vi "log analysis_gps.vi"() -> ()   [LabVIEW 2018] (continued)
\n\t\n15:48:12.2\tlog_raw\tgps_raw\t\tsystem status\tnormal 2 27.700000 0 0\trobot status\t93.017900\t121.985005\t8.053800\t-0.255095\t0.011947\t-127.616619\t0.344000\t0.011000\n\t\n15:48:12.7\tlog_raw\tgps_raw\t\tsystem status\tnormal 2 27.700000 0 0\trobot status\t92.936548\t121.892392\t8.053400\t-0.560051\t-0.370997\t-128.619129\t0.179000\t-0.036000\n\t\n15:48:13.2\tlog_raw\tgps_raw\t\tsystem status\tnormal 2 27.600000 0 0\trobot status\t92.838145\t121.787255\t8.053000\t-0.462743\t-0.497171\t-129.892844\t0.237000\t-0.153000\n\t\n15:48:13.7\tlog_raw\tgps_raw\t#INSPVAXA,USB3,0,46.5,FINESTEERING,2107,283711.750,02000000,471d,15824;INS_ALIGNMENT_COMPLETE,INS_RTKFIXED,37.37122661325,126.72188206330,8.0523,22.3000,-0.1946,-0.1990,0.0081,-0.343732019,-0.465256456,221.217414786,0.4342,0.3030,0.5793,0.1138,0.0937,0.0785,0.0954,0.0993,5.0883,0f000001,0*d2ab07a9\n\tsystem status\tnormal 2 27.600000 0 0\trobot status\t92.737843\t121.684862\t8.052300\t-0.343732\t-0.465256\t-131.217415\t0.296000\t-0.048000\n\t\n15:48:14.2\tlog_raw\tgps_raw\t#INSPVAXA,USB3,0,44.5,FINESTEERING,2107,283712.250,02000000,471d,15824;INS_ALIGNMENT_COMPLETE,INS_RTKFIXED,37.37122571809,126.72188087797,8.0513,22.3000,-0.1877,-0.2276,0.0316,0.179753839,-0.491470448,222.605830014,0.4342,0.3024,0.5794,0.1134,0.0940,0.0785,0.0954,0.0992,5.0887,0f000001,0*82158439\n\tsystem status\tnormal 2 27.500000 0 0\trobot status\t92.632849\t121.585514\t8.051300\t0.179754\t-0.491470\t-132.605830\t0.302000\t-0.060000\n\t\n15:48:14.7\tlog_raw\tgps_raw\t\tsystem status\tnormal 2 27.500000 0 0\trobot status\t92.530950\t121.487165\t8.046000\t-0.221044\t-0.411824\t-134.007632\t0.276000\t-0.043000\n\t\n15:48:15.2\tlog_raw\tgps_raw\t\tsystem status\tnormal 2 27.600000 0 0\trobot status\t92.422232\t121.387491\t8.042500\t-0.513663\t-0.512668\t-135.162406\t0.345000\t0.039000\n\t\n15:48:15.7\tlog_raw\tgps_raw\t\tsystem status\tnormal 2 27.600000 0 0\trobot status\t92.311835\t121.294033\t8.039900\t-0.332842\t-0.481399\t-136.078923\t0.343000\t0.036000\n\t\n15:48:16.2\tlog_raw\tgps_raw\t\tsystem status\tnormal 2 27.700000 0 0\trobot status\t92.199321\t121.200404\t8.038800\t-0.246424\t-0.569738\t-136.851756\t0.285000\t-0.056000\n\t\n15:48:16.7\tlog_raw\tgps_raw\t\tsystem status\tnormal 2 27.700000 0 0\trobot status\t92.091706\t121.109962\t8.035500\t-0.515195\t-0.354482\t-137.596544\t0.302000\t0.015000\n\t\n15:48:17.2\tlog_raw\tgps_raw\t\tsystem status\tnormal 2 27.800000 0 0\trobot status\t91.984102\t121.023401\t8.032900\t-0.648117\t-0.096859\t-138.155271\t0.305000\t0.062000\n\t\n15:48:17.7\tlog_raw\tgps_raw\t#INSPVAXA,USB3,0,49.5,FINESTEERING,2107,283715.750,02000000,471d,15824;INS_ALIGNMENT_COMPLETE,INS_RTKFIXED,37.37122004093,126.72187255202,8.0310,22.3000,-0.2525,-0.3284,0.0150,-0.722312377,-0.111566034,228.459144624,0.4339,0.3022,0.5793,0.1124,0.0928,0.0785,0.0954,0.0992,5.0842,0f000001,0*1d534d62\n\tsystem status\tnormal 2 27.700000 0 0\trobot status\t91.895350\t120.955445\t8.031000\t-0.722312\t-0.111566\t-138.459145\t0.356000\t0.005000\n\t\n15:48:18.2\tlog_raw\tgps_raw\t\tsystem status\tnormal 2 27.800000 0 0\trobot status\t91.784347\t120.867609\t8.027400\t-0.870891\t-0.276065\t-138.775579\t0.323000\t0.011000\n\t\n15:48:18.7\tlog_raw\tgps_raw\t\tsystem status\tnormal 2 27.800000 0 0\trobot status\t91.667786\t120.777478\t8.023500\t-0.860571\t-0.105772\t-139.137030\t0.415000\t0.024000\n\t\n15:48:19.2\tlog_raw\tgps_raw\t\tsystem status\tnormal 2 27.800000 0 0\trobot status\t91.467289\t120.615612\t8.019000\t-1.126128\t-0.570366\t-139.574346\t0.506000\t0.026000\n\t\n15:48:19.7\tlog_raw\tgps_raw\t\tsystem status\tnormal 2 27.900000 0 0\trobot status\t91.290630\t120.476156\t8.013000\t-1.186175\t-0.952521\t-139.872615\t0.485000\t0.025000\n\t\n15:48:20.2\tlog_raw\tgps_raw\t\tsystem status\tnormal 2 27.800000 0 0\trobot status\t91.107922\t120.338579\t8.010700\t-0.902776\t-1.033275\t-140.087143\t0.506000\t0.009000\n\t\n15:48:20.7\tlog_raw\tgps_raw\t\tsystem status\tnormal 2 27.800000 0 0\trobot status\t90.917995\t120.193959\t8.006900\t-1.049748\t-0.623872\t-140.229198\t0.504000\t0.022000\n\t\n15:48:21.2\tlog_raw\tgps_raw\t\tsystem status\tnormal 2 27.800000 0 0\trobot status\t90.727645\t120.053075\t8.003300\t-1.012052\t-0.230090\t-140.363200\t0.489000\t0.034000\n\t\n15:48:21.7\tlog_raw\tgps_raw\t\tsystem status\tnormal 2 27.800000 0 0\trobot status\t90.535348\t119.912993\t8.001800\t-0.988290\t-0.249157\t-140.250323\t0.490000\t0.034000\n\t\n15:48:22.2\tlog_raw\tgps_raw\t\tsystem status\tnormal 2 27.800000 0 0\trobot status\t90.365162\t119.792234\t7.999800\t-0.881256\t-0.195383\t-140.162244\t0.439000\t-0.029000\n\t\n15:48:22.7\tlog_raw\tgps_raw\t\tsystem status\tnormal 2 27.700000 0 0\trobot status\t90.166459\t119.645467\t7.997200\t-0.990730\t-0.386708\t-139.693095\t0.448000\t0.064000\n\t\n15:48:23.2\tlog_raw\tgps_raw\t\tsystem status\tnormal 2 27.600000 0 0\trobot status\t89.980110\t119.505285\t7.995900\t-0.920399\t-0.411056\t-138.884517\t0.331000\t0.293000\n\t\n15:48:23.7\tlog_raw\tgps_raw\t\tsystem status\tnormal 2 27.500000 0 0\trobot status\t89.798925\t119.364391\t7.991900\t-0.934473\t-0.125823\t-137.685217\t0.780000\t-0.350000\n\t\n15:48:24.3\tlog_raw\tgps_raw\t\tsystem status\tnormal 2 27.500000 0 0\trobot status\t89.618396\t119.217719\t7.990900\t-0.955434\t-0.178314\t-136.420655\t0.729000\t-0.315000\n\t\n15:48:24.8\tlog_raw\tgps_raw\t\tsystem status\tnormal 2 27.500000 0 0\trobot status\t89.438061\t119.065932\t7.990300\t-0.897105\t-0.363562\t-134.936703\t0.627000\t-0.123000\n\t\n15:48:25.3\tlog_raw\tgps_raw\t\tsystem status\tnormal 2 27.500000 0 0\trobot status\t89.259742\t118.908481\t7.988300\t-0.702072\t-0.768658\t-133.619038\t0.555000\t-0.042000\n\t\n15:48:25.8\tlog_raw\tgps_raw\t\tsystem status\tnormal 2 27.500000 0 0\trobot status\t89.085735\t118.748193\t7.985800\t-0.541349\t-0.915935\t-132.332460\t0.561000\t-0.086000\n\t\n15:48:26.3\tlog_raw\tgps_raw\t\tsystem status\tnormal 2 27.500000 0 0\trobot status\t88.921991\t118.588618\t7.982500\t-0.622601\t-0.502395\t-131.080219\t0.355000\t0.255000\n\t\n15:48:26.8\tlog_raw\tgps_raw\t\tsystem status\tnormal 2 27.500000 0 0\trobot status\t88.757318\t118.422538\t7.979600\t-0.531381\t-0.385527\t-129.950730\t0.648000\t-0.197000\n\t\n15:48:27.3\tlog_raw\tgps_raw\t\tsystem status\tnormal 2 27.500000 0 0\trobot status\t88.594631\t118.254427\t7.977200\t-0.446190\t-0.411819\t-128.968277\t0.666000\t-0.210000\n\t\n15:48:27.8\tlog_raw\tgps_raw\t\tsystem status\tnormal 2 27.600000 0 0\trobot status\t88.436524\t118.081442\t7.976100\t-0.854908\t-0.480169\t-128.206928\t0.457000\t0.071000\n\t\n15:48:28.3\tlog_raw\tgps_raw\t\tsystem status\tnormal 2 27.600000 0 0\trobot status\t88.280978\t117.911050\t7.973300\t-0.840223\t-0.485683\t-127.350658\t0.578000\t-0.111000\n\t\n15:48:28.8\tlog_raw\tgps_raw\t\tsystem status\tnormal 2 27.600000 0 0\trobot status\t88.125157\t117.734701\t7.973300\t-0.975629\t-0.460087\t-126.734726\t0.581000\t-0.092000\n\t\n15:48:29.3\tlog_raw\tgps_raw\t\tsystem status\tnormal 2 27.700000 0 0\trobot status\t87.972781\t117.556566\t7.972400\t-1.249899\t-0.684709\t-126.312420\t0.395000\t0.153000\n\t\n15:48:29.8\tlog_raw\tgps_raw\t\tsystem status\tnormal 2 27.700000 0 0\trobot status\t87.818562\t117.377164\t7.971600\t-1.130025\t-0.574230\t-125.881307\t0.422000\t0.152000\n\t\n15:48:30.3\tlog_raw\tgps_raw\t\tsystem status\tnormal 2 27.700000 0 0\trobot status\t87.670351\t117.200299\t7.971700\t-1.245931\t-0.391971\t-125.531082\t0.668000\t-0.259000\n\t\n15:48:30.8\tlog_raw\tgps_raw\t\tsystem status\tnormal 2 27.700000 0 0\trobot status\t87.521983\t117.020319\t7.971300\t-1.373248\t0.023524\t-125.204569\t0.362000\t0.195000\n\t\n15:48:31.3\tlog_raw\tgps_raw\t\tsystem status\tnormal 2 27.700000 0 0\trobot status\t87.374479\t116.840408\t7.972200\t-1.262386\t0.158447\t-124.787590\t0.497000\t0.002000\n\t\n15:48:31.8\tlog_raw\tgps_raw\t\tsystem status\tnormal 2 27.700000 0 0\trobot status\t87.236829\t116.671092\t7.974200\t-1.228214\t0.108580\t-124.545435\t0.542000\t0.007000\n\t\n15:48:32.3\tlog_raw\tgps_raw\t\tsystem status\tnormal 2 27.700000 0 0\trobot status\t87.089765\t116.488767\t7.975900\t-1.256331\t-0.129864\t-124.336401\t0.483000\t0.032000\n\t\n15:48:32.8\tlog_raw\tgps_raw\t\tsystem status\tnormal 2 27.700000 0 0\trobot status\t86.942897\t116.305166\t7.980600\t-1.436628\t0.013062\t-124.042497\t0.592000\t-0.138000\n\t\n15:48:33.3\tlog_raw\tgps_raw\t\tsystem status\tnormal 2 27.700000 0 0\trobot status\t86.791583\t116.117809\t7.982400\t-1.131604\t-0.146521\t-123.890554\t0.459000\t0.013000\n\t\n15:48:33.8\tlog_raw\tgps_raw\t#INSPVAXA,USB3,0,50.0,FINESTEERING,2107,283731.800,02000000,471d,15824;INS_ALIGNMENT_COMPLETE,INS_RTKFIXED,37.37117458679,126.72181307353,7.9818,22.3000,-0.3273,-0.2857,0.0109,-1.190065034,-0.069687290,213.721334289,0.4352,0.3028,0.5840,0.1128,0.0931,0.0809,0.0959,0.1000,5.0570,0f000001,0*9dfc8b18\n\tsystem status\tnormal 2 27.700000 0 0\trobot status\t86.626842\t115.910791\t7.981800\t-1.190065\t-0.069687\t-123.721334\t0.413000\t0.130000\n\t\n15:48:34.3\tlog_raw\tgps_raw\t\tsystem status\tnormal 2 27.800000 0 0\trobot status\t86.494276\t115.741589\t7.984700\t-1.380691\t-0.163770\t-123.599724\t0.490000\t0.027000\n\t\n15:48:34.8\tlog_raw\tgps_raw\t#INSPVAXA,USB3,0,51.0,FINESTEERING,2107,283732.800,02000000,471d,15824;INS_ALIGNMENT_COMPLETE,INS_RTKFIXED,37.37117121797,126.72180974634,7.9878,22.3000,-0.3313,-0.2857,0.0219,-1.270635454,-0.215524516,213.339771314,0.4352,0.3028,0.5846,0.1129,0.0933,0.0811,0.0960,0.1001,5.0551,0f000001,0*0aee9a35\n\tsystem status\tnormal 2 27.700000 0 0\trobot status\t86.332125\t115.536907\t7.987800\t-1.270635\t-0.215525\t-123.339771\t0.555000\t-0.092000\n\t\n15:48:35.3\tlog_raw\tgps_raw\t#INSPVAXA,USB3,0,51.5,FINESTEERING,2107,283733.300,02000000,471d,15824;INS_ALIGNMENT_COMPLETE,INS_RTKFIXED,37.37116954427,126.72180813326,7.9908,22.3000,-0.3552,-0.2859,0.0156,-1.448481440,-0.233169639,213.103409582,0.4350,0.3026,0.5849,0.1127,0.0932,0.0807,0.0961,0.1001,5.0540,0f000001,0*6eded770\n\tsystem status\tnormal 2 27.700000 0 0\trobot status\t86.189241\t115.351153\t7.990800\t-1.448481\t-0.233170\t-123.103410\t0.418000\t0.134000\n\t\n15:48:35.8\tlog_raw\tgps_raw\t\tsystem status\tnormal 2 27.700000 0 0\trobot status\t86.059476\t115.180486\t7.992600\t-1.482871\t-0.440891\t-122.862305\t0.381000\t0.175000\n\t\n15:48:36.3\tlog_raw\tgps_raw\t#INSPVAXA,USB3,0,50.5,FINESTEERING,2107,283734.300,02000000,471d,15824;INS_ALIGNMENT_COMPLETE,INS_RTKFIXED,37.37116643278,126.72180513242,7.9941,22.3000,-0.3478,-0.2920,-0.0081,-1.453049667,-0.445591431,212.491210472,0.4347,0.3023,0.5850,0.1126,0.0932,0.0804,0.0961,0.1001,5.0539,0f000001,0*79c2ad3a\n\tsystem status\tnormal 2 27.700000 0 0\trobot status\t85.923432\t115.005828\t7.994100\t-1.453050\t-0.445591\t-122.491210\t0.407000\t0.062000\n\t\n15:48:36.8\tlog_raw\tgps_raw\t\tsystem status\tnormal 2 27.700000 0 0\trobot status\t85.785092\t114.822258\t7.996500\t-1.200019\t-0.747046\t-122.371203\t0.383000\t0.098000\n\t\n15:48:37.3\tlog_raw\tgps_raw\t\tsystem status\tnormal 2 27.800000 0 0\trobot status\t85.644286\t114.630005\t7.999900\t-1.162405\t-0.500187\t-122.112655\t0.546000\t-0.078000\n\t\n15:48:37.8\tlog_raw\tgps_raw\t#INSPVAXA,USB3,0,50.0,FINESTEERING,2107,283735.800,02000000,471d,15824;INS_ALIGNMENT_COMPLETE,INS_RTKFIXED,37.37116119506,126.72180032977,8.0024,22.3000,-0.3542,-0.2959,0.0116,-1.070253035,-0.077101790,211.926024212,0.4346,0.3023,0.5850,0.1127,0.0933,0.0801,0.0962,0.1001,5.0543,0f000001,0*c680b455\n\tsystem status\tnormal 2 27.700000 0 0\trobot status\t85.498021\t114.424526\t8.002400\t-1.070253\t-0.077102\t-121.926024\t0.603000\t-0.154000\n\t\n15:48:38.3\tlog_raw\tgps_raw\t#INSPVAXA,USB3,0,52.5,FINESTEERING,2107,283736.300,02000000,471d,15824;INS_ALIGNMENT_COMPLETE,INS_RTKFIXED,37.37115947932,126.72179880714,8.0040,22.3000,-0.3644,-0.2930,0.0272,-1.158322238,-0.026079764,211.769815237,0.4340,0.3014,0.5849,0.1129,0.0936,0.0802,0.0962,0.1001,5.0557,0f000001,0*91878766\n\tsystem status\tnormal 2 27.700000 0 0\trobot status\t85.363149\t114.234107\t8.004000\t-1.158322\t-0.026080\t-121.769815\t0.444000\t0.091000\n\t\n15:48:38.8\tlog_raw\tgps_raw\t\tsystem status\tnormal 2 27.700000 0 0\trobot status\t85.241349\t114.062655\t8.007800\t-1.147952\t0.031214\t-121.613966\t0.431000\t0.095000\n\t\n15:48:39.3\tlog_raw\tgps_raw\t#INSPVAXA,USB3,0,49.5,FINESTEERING,2107,283737.300,02000000,471d,15824;INS_ALIGNMENT_COMPLETE,INS_RTKFIXED,37.37115601705,126.72179575213,8.0111,22.3000,-0.3535,-0.2715,0.0236,-1.072991275,-0.157444358,211.337264747,0.4338,0.3020,0.5848,0.1128,0.0935,0.0799,0.0962,0.1000,5.0571,0f000001,0*fcfec35c\n\tsystem status\tnormal 2 27.700000 0 0\trobot status\t85.092541\t113.849851\t8.011100\t-1.072991\t-0.157444\t-121.337265\t0.639000\t-0.209000\n\t\n15:48:39.8\tlog_raw\tgps_raw\t#INSPVAXA,USB3,0,49.5,FINESTEERING,2107,283737.800,02000000,471d,15824;INS_ALIGNMENT_COMPLETE,INS_RTKFIXED,37.37115424403,126.72179422575,8.0146,22.3000,-0.3686,-0.2725,0.0313,-1.104138059,-0.177331016,211.359293731,0.4338,0.3020,0.5848,0.1128,0.0935,0.0799,0.0962,0.1000,5.0571,0f000001,0*ab5647ea\n\tsystem status\tnormal 2 27.800000 0 0\trobot status\t84.957337\t113.653075\t8.014600\t-1.104138\t-0.177331\t-121.359294\t0.430000\t0.099000\n\t\n15:48:40.3\tlog_raw\tgps_raw\t\tsystem status\tnormal 2 27.700000 0 0\trobot status\t84.838628\t113.477755\t8.016900\t-1.353747\t-0.132621\t-121.323522\t0.573000\t-0.118000\n\t\n15:48:40.8\tlog_raw\tgps_raw\t\tsystem status\tnormal 2 27.800000 0 0\trobot status\t84.707094\t113.291580\t8.018800\t-1.250301\t-0.380341\t-121.163525\t0.339000\t-0.018000\n\t\n15:48:41.3\tlog_raw\tgps_raw\t#INSPVAXA,USB3,0,49.5,FINESTEERING,2107,283739.300,02000000,471d,15824;INS_ALIGNMENT_COMPLETE,INS_RTKFIXED,37.37114934907,126.72178999234,8.0211,22.3000,-0.4739,-0.3464,0.0176,-1.136581936,-0.167253224,210.967892029,0.4333,0.3019,0.5842,0.1128,0.0941,0.0795,0.0961,0.1000,5.0600,0f000001,0*70943433\n\tsystem status\tnormal 2 27.700000 0 0\trobot status\t84.582348\t113.109813\t8.021100\t-1.136582\t-0.167253\t-120.967892\t0.521000\t0.039000\n\t\n15:48:41.8\tlog_raw\tgps_raw\t\tsystem status\tnormal 2 27.800000 0 0\trobot status\t84.470112\t112.943563\t8.022300\t-1.050765\t-0.308716\t-120.878935\t0.430000\t0.006000\n\t\n15:48:42.3\tlog_raw\tgps_raw\t\tsystem status\tnormal 2 27.800000 0 0\trobot status\t84.332743\t112.735829\t8.022200\t-1.089765\t-0.132879\t-120.991930\t0.485000\t0.008000\n\t\n15:48:42.8\tlog_raw\tgps_raw\t#INSPVAXA,USB3,0,50.0,FINESTEERING,2107,283740.800,02000000,471d,15824;INS_ALIGNMENT_COMPLETE,INS_RTKFIXED,37.37114414583,126.72178561946,8.0225,22.3000,-0.3822,-0.2779,0.0042,-1.093019003,-0.010151528,210.947598498,0.4332,0.3033,0.5839,0.1127,0.0932,0.0793,0.0961,0.0999,5.0603,0f000001,0*1136f991\n\tsystem status\tnormal 2 27.700000 0 0\trobot status\t84.195006\t112.532337\t8.022500\t-1.093019\t-0.010152\t-120.947598\t0.504000\t0.001000\n\t\n15:48:43.3\tlog_raw\tgps_raw\t\tsystem status\tnormal 2 27.800000 0 0\trobot status\t84.075902\t112.352166\t8.023600\t-1.338722\t-0.304524\t-121.104447\t0.480000\t-0.009000\n\t\n15:48:43.8\tlog_raw\tgps_raw\t#INSPVAXA,USB3,0,48.5,FINESTEERING,2107,283741.800,02000000,471d,15824;INS_ALIGNMENT_COMPLETE,INS_RTKFIXED,37.37114058594,126.72178265531,8.0253,22.3000,-0.3567,-0.2593,0.0215,-1.513936100,-0.057286463,211.372668569,0.4332,0.3024,0.5836,0.1132,0.0938,0.0801,0.0960,0.0999,5.0615,0f000001,0*2f761fac\n\tsystem status\tnormal 2 27.800000 0 0\trobot status\t83.932446\t112.137247\t8.025300\t-1.513936\t-0.057286\t-121.372669\t0.502000\t-0.009000\n\t\n15:48:44.3\tlog_raw\tgps_raw\t#INSPVAXA,USB3,0,48.5,FINESTEERING,2107,283742.300,02000000,471d,15824;INS_ALIGNMENT_COMPLETE,INS_RTKFIXED,37.37113883610,126.72178116483,8.0251,22.3000,-0.3566,-0.2646,-0.0002,-1.629553261,-0.371874785,211.544863069,0.4334,0.3022,0.5834,0.1130,0.0935,0.0799,0.0960,0.0999,5.0629,0f000001,0*db798f34\n\tsystem status\tnormal 2 27.800000 0 0\trobot status\t83.800422\t111.943043\t8.025100\t-1.629553\t-0.371875\t-121.544863\t0.489000\t-0.014000\n\t\n15:48:44.8\tlog_raw\tgps_raw\t#INSPVAXA,USB3,0,48.5,FINESTEERING,2107,283742.800,02000000,471d,15824;INS_ALIGNMENT_COMPLETE,INS_RTKFIXED,37.37113713184,126.72177968059,8.0243,22.3000,-0.3489,-0.2579,0.0216,-1.473854332,-0.365287327,211.722184950,0.4334,0.3022,0.5834,0.1130,0.0935,0.0799,0.0960,0.0999,5.0629,0f000001,0*7daa81b7\n\tsystem status\tnormal 2 27.800000 0 0\trobot status\t83.668950\t111.753898\t8.024300\t-1.473854\t-0.365287\t-121.722185\t0.486000\t-0.016000\n\t\n15:48:45.3\tlog_raw\tgps_raw\t#INSPVAXA,USB3,0,46.0,FINESTEERING,2107,283743.300,02000000,471d,15824;INS_ALIGNMENT_COMPLETE,INS_RTKFIXED,37.37113541318,126.72177817924,8.0241,22.3000,-0.3602,-0.2594,0.0280,-1.547897785,-0.197369444,211.857866163,0.4337,0.3019,0.5833,0.1132,0.0937,0.0803,0.0960,0.0999,5.0644,0f000001,0*9acc447f\n\tsystem status\tnormal 2 27.800000 0 0\trobot status\t83.535963\t111.563154\t8.024100\t-1.547898\t-0.197369\t-121.857866\t0.490000\t-0.018000\n\t\n15:48:45.8\tlog_raw\tgps_raw\t#INSPVAXA,USB3,0,46.0,FINESTEERING,2107,283743.800,02000000,471d,15824;INS_ALIGNMENT_COMPLETE,INS_RTKFIXED,37.37113371860,126.72177667415,8.0236,22.3000,-0.3426,-0.2605,-0.0024,-1.484785571,-0.050192547,211.992358658,0.4337,0.3019,0.5833,0.1132,0.0937,0.0803,0.0960,0.0999,5.0644,0f000001,0*53a396a3\n\tsystem status\tnormal 2 27.800000 0 0\trobot status\t83.402645\t111.375083\t8.023600\t-1.484786\t-0.050193\t-121.992359\t0.494000\t-0.016000\n\t\n15:48:46.3\tlog_raw\tgps_raw\t#INSPVAXA,USB3,0,49.5,FINESTEERING,2107,283744.300,02000000,471d,15824;INS_ALIGNMENT_COMPLETE,INS_RTKFIXED,37.37113201879,126.72177513465,8.0232,22.3000,-0.3446,-0.2615,0.0259,-1.383371091,0.074969047,212.298273108,0.4337,0.3020,0.5833,0.1129,0.0934,0.0801,0.0960,0.0999,5.0660,0f000001,0*aa113718\n\tsystem status\tnormal 2 27.800000 0 0\trobot status\t83.266279\t111.186432\t8.023200\t-1.383371\t0.074969\t-122.298273\t0.499000\t-0.007000\n\t\n15:48:46.8\tlog_raw\tgps_raw\t#INSPVAXA,USB3,0,49.5,FINESTEERING,2107,283744.800,02000000,471d,15824;INS_ALIGNMENT_COMPLETE,INS_RTKFIXED,37.37113032635,126.72177358354,8.0234,22.3000,-0.3375,-0.2772,0.0273,-1.329281946,0.043160679,212.609113265,0.4337,0.3020,0.5833,0.1129,0.0934,0.0801,0.0960,0.0999,5.0660,0f000001,0*0ee78c5b\n\tsystem status\tnormal 2 27.800000 0 0\trobot status\t83.128884\t110.998599\t8.023400\t-1.329282\t0.043161\t-122.609113\t0.489000\t-0.016000\n\t\n15:48:47.3\tlog_raw\tgps_raw\t#INSPVAXA,USB3,0,52.0,FINESTEERING,2107,283745.300,02000000,471d,15824;INS_ALIGNMENT_COMPLETE,INS_RTKFIXED,37.37112862779,126.72177199929,8.0231,22.3000,-0.3459,-0.2782,0.0216,-1.184506207,0.212511857,212.764446314,0.4334,0.3022,0.5833,0.1126,0.0933,0.0799,0.0960,0.0999,5.0673,0f000001,0*6b47a2c0\n\tsystem status\tnormal 2 27.800000 0 0\trobot status\t82.988553\t110.810086\t8.023100\t-1.184506\t0.212512\t-122.764446\t0.506000\t-0.008000\n\t\n15:48:47.8\tlog_raw\tgps_raw\t\tsystem status\tnormal 2 27.800000 0 0\trobot status\t82.860769\t110.640040\t8.024500\t-1.218748\t0.257104\t-123.000230\t0.493000\t-0.007000\n\t\n15:48:48.3\tlog_raw\tgps_raw\t#INSPVAXA,USB3,0,50.5,FINESTEERING,2107,283746.300,02000000,471d,15824;INS_ALIGNMENT_COMPLETE,INS_RTKFIXED,37.37112521282,126.72176875566,8.0246,22.3000,-0.3436,-0.2866,0.0107,-1.152398634,0.173487967,213.302028541,0.4332,0.3024,0.5833,0.1125,0.0932,0.0797,0.0960,0.0999,5.0684,0f000001,0*49aabec8\n\tsystem status\tnormal 2 27.800000 0 0\trobot status\t82.701238\t110.431080\t8.024600\t-1.152399\t0.173488\t-123.302029\t0.485000\t-0.005000\n\t\n15:48:48.8\tlog_raw\tgps_raw\t#INSPVAXA,USB3,0,50.5,FINESTEERING,2107,283746.800,02000000,471d,15824;INS_ALIGNMENT_COMPLETE,INS_RTKFIXED,37.37112349330,126.72176709470,8.0242,22.3000,-0.3497,-0.2797,0.0191,-1.314916766,0.110853537,213.600359109,0.4332,0.3024,0.5833,0.1125,0.0932,0.0797,0.0960,0.0999,5.0684,0f000001,0*7436a872\n\tsystem status\tnormal 2 27.800000 0 0\trobot status\t82.554113\t110.240241\t8.024200\t-1.314917\t0.110854\t-123.600359\t0.500000\t-0.013000\n\t\n15:48:49.3\tlog_raw\tgps_raw\t#INSPVAXA,USB3,0,49.0,FINESTEERING,2107,283747.300,02000000,471d,15824;INS_ALIGNMENT_COMPLETE,INS_RTKFIXED,37.37112180863,126.72176542630,8.0244,22.3000,-0.3486,-0.2973,0.0020,-1.259459400,-0.205839817,213.873121305,0.4330,0.3028,0.5834,0.1123,0.0929,0.0795,0.0961,0.0999,5.0687,0f000001,0*73ffb7ee\n\tsystem status\tnormal 2 27.800000 0 0\trobot status\t82.406329\t110.053270\t8.024400\t-1.259459\t-0.205840\t-123.873121\t0.501000\t-0.018000\n\t\n15:48:49.8\tlog_raw\tgps_raw\t#INSPVAXA,USB3,0,49.0,FINESTEERING,2107,283747.800,02000000,471d,15824;INS_ALIGNMENT_COMPLETE,INS_RTKFIXED,37.37112013539,126.72176372884,8.0242,22.3000,-0.3447,-0.2936,0.0201,-1.219688710,-0.227511135,214.058949387,0.4330,0.3028,0.5834,0.1123,0.0929,0.0795,0.0961,0.0999,5.0687,0f000001,0*4b57b427\n\tsystem status\tnormal 2 27.800000 0 0\trobot status\t82.255971\t109.867567\t8.024200\t-1.219689\t-0.227511\t-124.058949\t0.493000\t-0.003000\n\t\n15:48:50.3\tlog_raw\tgps_raw\t\tsystem status\tnormal 2 27.800000 0 0\trobot status\t82.125100\t109.705360\t8.022900\t-1.272959\t-0.391336\t-124.294640\t0.474000\t0.015000\n\t\n15:48:50.8\tlog_raw\tgps_raw\t#INSPVAXA,USB3,0,51.0,FINESTEERING,2107,283748.800,02000000,471d,15824;INS_ALIGNMENT_COMPLETE,INS_RTKFIXED,37.37111693523,126.72176047327,8.0217,22.3000,-0.3794,-0.3424,0.0221,-1.127145988,-0.211560747,214.369143208,0.4328,0.3022,0.5832,0.1125,0.0931,0.0797,0.0961,0.0999,5.0695,0f000001,0*f768fbb4\n\tsystem status\tnormal 2 27.800000 0 0\trobot status\t81.967598\t109.512402\t8.021700\t-1.127146\t-0.211561\t-124.369143\t0.521000\t0.000000\n\t\n15:48:51.3\tlog_raw\tgps_raw\t#INSPVAXA,USB3,0,48.0,FINESTEERING,2107,283749.300,02000000,471d,15824;INS_ALIGNMENT_COMPLETE,INS_RTKFIXED,37.37111528295,126.72175880850,8.0228,22.3000,-0.3091,-0.2843,0.0017,-1.226699576,0.077786636,214.515601245,0.4326,0.3019,0.5831,0.1128,0.0935,0.0801,0.0961,0.1000,5.0707,0f000001,0*33e38593\n\tsystem status\tnormal 2 27.800000 0 0\trobot status\t81.820135\t109.329026\t8.022800\t-1.226700\t0.077787\t-124.515601\t0.481000\t-0.012000\n\t\n15:48:51.8\tlog_raw\tgps_raw\t#INSPVAXA,USB3,0,48.0,FINESTEERING,2107,283749.800,02000000,471d,15824;INS_ALIGNMENT_COMPLETE,INS_RTKFIXED,37.37111354772,126.72175702907,8.0230,22.3000,-0.3442,-0.3142,0.0177,-1.011041502,-0.010822308,214.650851385,0.4326,0.3019,0.5831,0.1128,0.0935,0.0801,0.0961,0.1000,5.0707,0f000001,0*157ce5bb\n\tsystem status\tnormal 2 27.800000 0 0\trobot status\t81.662516\t109.136443\t8.023000\t-1.011042\t-0.010822\t-124.650851\t0.501000\t0.006000\n\t\n15:48:52.3\tlog_raw\tgps_raw\t\tsystem status\tnormal 2 27.800000 0 0\trobot status\t81.529444\t108.971054\t8.023600\t-1.134131\t-0.000127\t-124.709887\t0.497000\t0.000000\n\t\n15:48:52.8\tlog_raw\tgps_raw\t\tsystem status\tnormal 2 27.800000 0 0\trobot status\t81.377778\t108.780675\t8.026800\t-1.391204\t-0.015262\t-124.810162\t0.496000\t0.005000\n\t\n15:48:53.3\tlog_raw\tgps_raw\t#INSPVAXA,USB3,0,50.0,FINESTEERING,2107,283751.300,02000000,471d,15824;INS_ALIGNMENT_COMPLETE,INS_RTKFIXED,37.37110849817,126.72175192105,8.0275,22.3000,-0.3358,-0.3126,0.0172,-1.035437411,0.273015584,214.819783864,0.4328,0.3018,0.5834,0.1129,0.0936,0.0806,0.0961,0.1000,5.0732,0f000001,0*f034d66d\n\tsystem status\tnormal 2 27.800000 0 0\trobot status\t81.210056\t108.576025\t8.027500\t-1.035437\t0.273016\t-124.819784\t0.503000\t-0.001000\n\t\n15:48:53.8\tlog_raw\tgps_raw\t#INSPVAXA,USB3,0,50.0,FINESTEERING,2107,283751.800,02000000,471d,15824;INS_ALIGNMENT_COMPLETE,INS_RTKFIXED,37.37110680705,126.72175019748,8.0301,22.3000,-0.3539,-0.3161,0.0213,-1.037720149,0.378523097,214.886319407,0.4328,0.3018,0.5834,0.1129,0.0936,0.0806,0.0961,0.1000,5.0732,0f000001,0*08748abc\n\tsystem status\tnormal 2 27.800000 0 0\trobot status\t81.057385\t108.388339\t8.030100\t-1.037720\t0.378523\t-124.886319\t0.505000\t-0.009000\n\t\n15:48:54.3\tlog_raw\tgps_raw\t#INSPVAXA,USB3,0,49.5,FINESTEERING,2107,283752.300,02000000,471d,15824;INS_ALIGNMENT_COMPLETE,INS_RTKFIXED,37.37110513951,126.72174852580,8.0342,22.3000,-0.3395,-0.3054,0.0275,-1.169969735,0.177564821,214.703949877,0.4330,0.3019,0.5837,0.1127,0.0933,0.0804,0.0962,0.1001,5.0745,0f000001,0*3b22e019\n\tsystem status\tnormal 2 27.800000 0 0\trobot status\t80.909310\t108.203269\t8.034200\t-1.169970\t0.177565\t-124.703950\t0.459000\t0.049000\n\t\n15:48:54.8\tlog_raw\tgps_raw\t#INSPVAXA,USB3,0,49.5,FINESTEERING,2107,283752.800,02000000,471d,15824;INS_ALIGNMENT_COMPLETE,INS_RTKFIXED,37.37110344707,126.72174683245,8.0372,22.3000,-0.3480,-0.3077,0.0306,-1.217859023,0.163695826,214.472427666,0.4330,0.3019,0.5837,0.1127,0.0933,0.0804,0.0962,0.1001,5.0745,0f000001,0*0f7f998b\n\tsystem status\tnormal 2 27.800000 0 0\trobot status\t80.759316\t108.015435\t8.037200\t-1.217859\t0.163696\t-124.472428\t0.575000\t-0.108000\n\t\n15:48:55.3\tlog_raw\tgps_raw\t#INSPVAXA,USB3,0,49.0,FINESTEERING,2107,283753.300,02000000,471d,15824;INS_ALIGNMENT_COMPLETE,INS_RTKFIXED,37.37110176276,126.72174513892,8.0405,22.3000,-0.3362,-0.2959,0.0055,-0.953272899,0.159929728,214.321717849,0.4329,0.3016,0.5838,0.1125,0.0931,0.0801,0.0962,0.1001,5.0760,0f000001,0*9e9621c6\n\tsystem status\tnormal 2 27.800000 0 0\trobot status\t80.609306\t107.828504\t8.040500\t-0.953273\t0.159930\t-124.321718\t0.468000\t0.046000\n\t\n15:48:55.8\tlog_raw\tgps_raw\t#INSPVAXA,USB3,0,49.0,FINESTEERING,2107,283753.800,02000000,471d,15824;INS_ALIGNMENT_COMPLETE,INS_RTKFIXED,37.37110008196,126.72174349775,8.0442,22.3000,-0.3613,-0.3106,0.0312,-1.166829812,0.116996203,214.014548565,0.4329,0.3016,0.5838,0.1125,0.0931,0.0801,0.0962,0.1001,5.0760,0f000001,0*f55bb199\n\tsystem status\tnormal 2 27.700000 0 0\trobot status\t80.463934\t107.641963\t8.044200\t-1.166830\t0.116996\t-124.014549\t0.471000\t0.050000\n\t\n15:48:56.3\tlog_raw\tgps_raw\t#INSPVAXA,USB3,0,50.5,FINESTEERING,2107,283754.300,02000000,471d,15824;INS_ALIGNMENT_COMPLETE,INS_RTKFIXED,37.37109836373,126.72174184574,8.0475,22.3000,-0.3327,-0.2951,0.0321,-1.340604372,0.249067491,213.619073128,0.4327,0.3010,0.5839,0.1123,0.0933,0.0799,0.0962,0.1001,5.0774,0f000001,0*1e6eecd6\n\tsystem status\tnormal 2 27.700000 0 0\trobot status\t80.317601\t107.451267\t8.047500\t-1.340604\t0.249067\t-123.619073\t0.436000\t0.095000\n\t\n15:48:56.8\tlog_raw\tgps_raw\t#INSPVAXA,USB3,0,50.5,FINESTEERING,2107,283754.800,02000000,471d,15824;INS_ALIGNMENT_COMPLETE,INS_RTKFIXED,37.37109667964,126.72174020389,8.0524,22.3000,-0.3499,-0.2857,0.0212,-1.089589442,0.349909054,213.310894710,0.4327,0.3010,0.5839,0.1123,0.0933,0.0799,0.0962,0.1001,5.0774,0f000001,0*4cfde7b0\n\tsystem status\tnormal 2 27.700000 0 0\trobot status\t80.172169\t107.264360\t8.052400\t-1.089589\t0.349909\t-123.310895\t0.429000\t0.123000\n\t\n15:48:57.3\tlog_raw\tgps_raw\t#INSPVAXA,USB3,0,50.0,FINESTEERING,2107,283755.300,02000000,471d,15824;INS_ALIGNMENT_COMPLETE,INS_RTKFIXED,37.37109494631,126.72173857933,8.0558,22.3000,-0.3482,-0.3112,0.0327,-1.123456133,0.254250073,212.973630812,0.4328,0.3002,0.5840,0.1125,0.0933,0.0800,0.0962,0.1002,5.0783,0f000001,0*6370c8f7\n\tsystem status\tnormal 2 27.800000 0 0\trobot status\t80.028268\t107.071989\t8.055800\t-1.123456\t0.254250\t-122.973631\t0.586000\t-0.136000\n\t\n15:48:57.8\tlog_raw\tgps_raw\t#INSPVAXA,USB3,0,50.0,FINESTEERING,2107,283755.800,02000000,471d,15824;INS_ALIGNMENT_COMPLETE,INS_RTKFIXED,37.37109323993,126.72173698484,8.0607,22.3000,-0.3643,-0.2927,0.0186,-1.115855413,0.320489035,212.665195189,0.4328,0.3002,0.5840,0.1125,0.0933,0.0800,0.0962,0.1002,5.0783,0f000001,0*79f1de9b\n\tsystem status\tnormal 2 27.700000 0 0\trobot status\t79.887031\t106.882608\t8.060700\t-1.115855\t0.320489\t-122.665195\t0.577000\t-0.116000\n\t\n15:48:58.3\tlog_raw\tgps_raw\t#INSPVAXA,USB3,0,49.0,FINESTEERING,2107,283756.300,02000000,471d,15824;INS_ALIGNMENT_COMPLETE,INS_RTKFIXED,37.37109147412,126.72173536418,8.0658,22.3000,-0.3720,-0.2998,0.0176,-0.967758336,0.009147585,212.513392073,0.4329,0.3001,0.5842,0.1131,0.0941,0.0808,0.0962,0.1002,5.0788,0f000001,0*480160b6\n\tsystem status\tnormal 2 27.700000 0 0\trobot status\t79.743475\t106.686632\t8.065800\t-0.967758\t0.009148\t-122.513392\t0.594000\t-0.134000\n\t\n15:48:58.8\tlog_raw\tgps_raw\t#INSPVAXA,USB3,0,49.0,FINESTEERING,2107,283756.800,02000000,471d,15824;INS_ALIGNMENT_COMPLETE,INS_RTKFIXED,37.37108975069,126.72173380065,8.0704,22.3000,-0.3560,-0.3018,0.0441,-0.888869342,0.191957925,212.381344702,0.4329,0.3001,0.5842,0.1131,0.0941,0.0808,0.0962,0.1002,5.0788,0f000001,0*35d96739\n\tsystem status\tnormal 2 27.700000 0 0\trobot status\t79.604981\t106.495359\t8.070400\t-0.888869\t0.191958\t-122.381345\t0.461000\t0.055000\n\t\n15:48:59.3\tlog_raw\tgps_raw\t#INSPVAXA,USB3,0,50.5,FINESTEERING,2107,283757.300,02000000,471d,15824;INS_ALIGNMENT_COMPLETE,INS_RTKFIXED,37.37108800138,126.72173224082,8.0747,22.3000,-0.3610,-0.2896,0.0115,-0.827433156,0.184771072,212.230918209,0.4331,0.3002,0.5847,0.1138,0.0947,0.0820,0.0961,0.1002,5.0788,0f000001,0*487ee94f\n\tsystem status\tnormal 2 27.800000 0 0\trobot status\t79.466813\t106.301214\t8.074700\t-0.827433\t0.184771\t-122.230918\t0.428000\t0.115000\n\t\n15:48:59.8\tlog_raw\tgps_raw\t#INSPVAXA,USB3,0,50.5,FINESTEERING,2107,283757.800,02000000,471d,15824;INS_ALIGNMENT_COMPLETE,INS_RTKFIXED,37.37108628681,126.72173070436,8.0804,22.3000,-0.3571,-0.2959,0.0231,-0.782297314,0.234364659,212.024110500,0.4331,0.3002,0.5847,0.1138,0.0947,0.0820,0.0961,0.1002,5.0788,0f000001,0*d45b12f8\n\tsystem status\tnormal 2 27.800000 0 0\trobot status\t79.330716\t106.110924\t8.080400\t-0.782297\t0.234365\t-122.024111\t0.539000\t-0.078000\n\t\n15:49:00.3\tlog_raw\tgps_raw\t#INSPVAXA,USB3,0,48.5,FINESTEERING,2107,283758.300,02000000,471d,15824;INS_ALIGNMENT_COMPLETE,INS_RTKFIXED,37.37108452216,126.72172915072,8.0875,22.3000,-0.3471,-0.2721,0.0431,-0.667161405,0.478660686,212.038204919,0.4334,0.3007,0.5852,0.1141,0.0949,0.0828,0.0961,0.1002,5.0790,0f000001,0*96971f51\n\tsystem status\tnormal 2 27.800000 0 0\trobot status\t79.193097\t105.915077\t8.087500\t-0.667161\t0.478661\t-122.038205\t0.475000\t0.003000\n\t\n15:49:00.8\tlog_raw\tgps_raw\t#INSPVAXA,USB3,0,48.5,FINESTEERING,2107,283758.800,02000000,471d,15824;INS_ALIGNMENT_COMPLETE,INS_RTKFIXED,37.37108279307,126.72172764103,8.0915,22.3000,-0.3762,-0.2924,0.0247,-0.558954729,0.708405130,211.994899529,0.4334,0.3007,0.5852,0.1141,0.0949,0.0828,0.0961,0.1002,5.0790,0f000001,0*cea2d680\n\tsystem status\tnormal 2 27.800000 0 0\trobot status\t79.059371\t105.723175\t8.091500\t-0.558955\t0.708405\t-121.994900\t0.502000\t-0.015000\n\t\n15:49:01.3\tlog_raw\tgps_raw\t#INSPVAXA,USB3,0,49.0,FINESTEERING,2107,283759.300,02000000,471d,15824;INS_ALIGNMENT_COMPLETE,INS_RTKFIXED,37.37108105868,126.72172613061,8.0959,22.3000,-0.3577,-0.2867,0.0280,-0.582378348,0.657248955,212.009317434,0.4336,0.3012,0.5858,0.1140,0.0947,0.0830,0.0962,0.1003,5.0797,0f000001,0*cc7fd0eb\n\tsystem status\tnormal 2 27.800000 0 0\trobot status\t78.925581\t105.530686\t8.095900\t-0.582378\t0.657249\t-122.009317\t0.481000\t0.018000\n\t\n15:49:01.8\tlog_raw\tgps_raw\t#INSPVAXA,USB3,0,49.0,FINESTEERING,2107,283759.800,02000000,471d,15824;INS_ALIGNMENT_COMPLETE,INS_RTKFIXED,37.37107931872,126.72172458410,8.1011,22.3000,-0.3599,-0.2848,0.0379,-0.459271249,0.431724641,212.075547686,0.4336,0.3012,0.5858,0.1140,0.0947,0.0830,0.0962,0.1003,5.0797,0f000001,0*b3831dc9\n\tsystem status\tnormal 2 27.800000 0 0\trobot status\t78.788594\t105.337579\t8.101100\t-0.459271\t0.431725\t-122.075548\t0.496000\t-0.003000\n\t\n15:49:02.3\tlog_raw\tgps_raw\t#INSPVAXA,USB3,0,49.0,FINESTEERING,2107,283760.300,02000000,471d,15824;INS_ALIGNMENT_COMPLETE,INS_RTKFIXED,37.37107757487,126.72172306983,8.1066,22.3000,-0.3662,-0.2801,0.0079,-0.623221926,0.408229344,212.074392228,0.4338,0.3017,0.5866,0.1138,0.0944,0.0831,0.0962,0.1003,5.0809,0f000001,0*d3997e6b\n\tsystem status\tnormal 2 27.800000 0 0\trobot status\t78.654462\t105.144039\t8.106600\t-0.623222\t0.408229\t-122.074392\t0.495000\t-0.002000\n\t\n15:49:02.8\tlog_raw\tgps_raw\t#INSPVAXA,USB3,0,49.0,FINESTEERING,2107,283760.800,02000000,471d,15824;INS_ALIGNMENT_COMPLETE,INS_RTKFIXED,37.37107585658,126.72172154929,8.1105,22.3000,-0.3559,-0.2976,0.0252,-0.619300370,0.317089157,212.125818977,0.4338,0.3017,0.5866,0.1138,0.0944,0.0831,0.0962,0.1003,5.0809,0f000001,0*2578c1d0\n\tsystem status\tnormal 2 27.800000 0 0\trobot status\t78.519775\t104.953337\t8.110500\t-0.619300\t0.317089\t-122.125819\t0.502000\t-0.005000\n\t\n15:49:03.3\tlog_raw\tgps_raw\t#INSPVAXA,USB3,0,47.5,FINESTEERING,2107,283761.300,02000000,471d,15824;INS_ALIGNMENT_COMPLETE,INS_RTKFIXED,37.37107412615,126.72172002171,8.1136,22.3000,-0.3598,-0.2783,0.0314,-0.587667385,0.123936522,212.281601914,0.4339,0.3017,0.5874,0.1136,0.0941,0.0830,0.0963,0.1004,5.0820,0f000001,0*f4eeef52\n\tsystem status\tnormal 2 27.800000 0 0\trobot status\t78.384465\t104.761287\t8.113600\t-0.587667\t0.123937\t-122.281602\t0.479000\t-0.020000\n\t\n15:49:03.8\tlog_raw\tgps_raw\t#INSPVAXA,USB3,0,47.5,FINESTEERING,2107,283761.800,02000000,471d,15824;INS_ALIGNMENT_COMPLETE,INS_RTKFIXED,37.37107239859,126.72171850723,8.1174,22.3000,-0.3618,-0.2694,0.0247,-0.806586304,0.185409278,212.363938082,0.4339,0.3017,0.5874,0.1136,0.0941,0.0830,0.0963,0.1004,5.0820,0f000001,0*fafaa8b9\n\tsystem status\tnormal 2 27.800000 0 0\trobot status\t78.250314\t104.569556\t8.117400\t-0.806586\t0.185409\t-122.363938\t0.497000\t-0.007000\n\t\n15:49:04.3\tlog_raw\tgps_raw\t#INSPVAXA,USB3,0,49.5,FINESTEERING,2107,283762.300,02000000,471d,15824;INS_ALIGNMENT_COMPLETE,INS_RTKFIXED,37.37107064339,126.72171694758,8.1181,22.3000,-0.3599,-0.2839,0.0222,-0.849299208,0.007344260,212.586929026,0.4338,0.3017,0.5881,0.1135,0.0943,0.0833,0.0964,0.1005,5.0831,0f000001,0*fde6b9b2\n\tsystem status\tnormal 2 27.800000 0 0\trobot status\t78.112163\t104.374757\t8.118100\t-0.849299\t0.007344\t-122.586929\t0.498000\t-0.003000\n\t\n15:49:04.8\tlog_raw\tgps_raw\t#DUALANTENNAHEADINGA,USB3,0,49.5,FINESTEERING,2107,283762.800,02000000,d426,15824;INSUFFICIENT_OBS,NONE,-1.000000000,0.000000000,0.000000000,0.0,0.000000000,0.000000000,\"631T\",11,2,2,2,04,00,20,00*344581c2\n\tsystem status\tnormal 2 27.800000 0 0\trobot status\t77.975232\t104.184643\t8.121000\t-0.904925\t-0.307789\t-122.786142\t0.488000\t-0.019000\n\t\n15:49:05.3\tlog_raw\tgps_raw\t#INSPVAXA,USB3,0,49.5,FINESTEERING,2107,283763.300,02000000,471d,15824;INS_ALIGNMENT_COMPLETE,INS_RTKFIXED,37.37106722577,126.72171383567,8.1242,22.3000,-0.3707,-0.2828,0.0344,-0.877287415,-0.329953157,212.884392391,0.4341,0.3014,0.5889,0.1138,0.0946,0.0836,0.0965,0.1006,5.0839,0f000001,0*2db501e2\n\tsystem status\tnormal 2 27.800000 0 0\trobot status\t77.836515\t103.995456\t8.124200\t-0.877287\t-0.329953\t-122.884392\t0.502000\t0.000000\n\t\n15:49:05.8\tlog_raw\tgps_raw\t#INSPVAXA,USB3,0,49.5,FINESTEERING,2107,283763.800,02000000,471d,15824;INS_ALIGNMENT_COMPLETE,INS_RTKFIXED,37.37106551581,126.72171225128,8.1242,22.3000,-0.3497,-0.2822,0.0044,-0.644975976,-0.227422020,213.086413848,0.4341,0.3014,0.5889,0.1138,0.0946,0.0836,0.0965,0.1006,5.0839,0f000001,0*e7a51fd5\n\tsystem status\tnormal 2 27.800000 0 0\trobot status\t77.696173\t103.805678\t8.124200\t-0.644976\t-0.227422\t-123.086414\t0.490000\t-0.007000\n\t\n15:49:06.3\tlog_raw\tgps_raw\t#INSPVAXA,USB3,0,50.0,FINESTEERING,2107,283764.300,02000000,471d,15824;INS_ALIGNMENT_COMPLETE,INS_RTKFIXED,37.37106379034,126.72171067271,8.1222,22.3000,-0.3531,-0.2829,0.0306,-0.817396197,-0.204433431,213.191870760,0.4344,0.3013,0.5897,0.1145,0.0953,0.0847,0.0966,0.1006,5.0845,0f000001,0*c35694b0\n\tsystem status\tnormal 2 27.800000 0 0\trobot status\t77.556345\t103.614179\t8.122200\t-0.817396\t-0.204433\t-123.191871\t0.487000\t-0.013000\n\t\n15:49:06.8\tlog_raw\tgps_raw\t#INSPVAXA,USB3,0,50.0,FINESTEERING,2107,283764.800,02000000,471d,15824;INS_ALIGNMENT_COMPLETE,INS_RTKFIXED,37.37106210013,126.72170911188,8.1232,22.3000,-0.3512,-0.2846,0.0354,-0.878103846,0.017122797,213.188721115,0.4344,0.3013,0.5897,0.1145,0.0953,0.0847,0.0966,0.1006,5.0845,0f000001,0*f1b4f4ee\n\tsystem status\tnormal 2 27.800000 0 0\trobot status\t77.418090\t103.426593\t8.123200\t-0.878104\t0.017123\t-123.188721\t0.498000\t0.003000\n\t\n15:49:07.3\tlog_raw\tgps_raw\t#INSPVAXA,USB3,0,48.5,FINESTEERING,2107,283765.300,02000000,471d,15824;INS_ALIGNMENT_COMPLETE,INS_RTKFIXED,37.37106036944,126.72170751159,8.1232,22.3000,-0.3518,-0.2906,0.0186,-0.822067301,0.160317962,213.455699651,0.4347,0.3015,0.5906,0.1149,0.0956,0.0855,0.0967,0.1007,5.0850,0f000001,0*76086230\n\tsystem status\tnormal 2 27.800000 0 0\trobot status\t77.276339\t103.234514\t8.123200\t-0.822067\t0.160318\t-123.455700\t0.490000\t-0.006000\n\t\n15:49:07.8\tlog_raw\tgps_raw\t#INSPVAXA,USB3,0,48.5,FINESTEERING,2107,283765.800,02000000,471d,15824;INS_ALIGNMENT_COMPLETE,INS_RTKFIXED,37.37105862901,126.72170591999,8.1228,22.3000,-0.3574,-0.2825,0.0115,-1.119312429,-0.040061536,213.743406523,0.4347,0.3015,0.5906,0.1149,0.0956,0.0855,0.0967,0.1007,5.0850,0f000001,0*ba4559e2\n\tsystem status\tnormal 2 27.800000 0 0\trobot status\t77.135357\t103.041355\t8.122800\t-1.119312\t-0.040062\t-123.743407\t0.492000\t-0.007000\n\t\n15:49:08.3\tlog_raw\tgps_raw\t#INSPVAXA,USB3,0,49.5,FINESTEERING,2107,283766.300,02000000,471d,15824;INS_ALIGNMENT_COMPLETE,INS_RTKFIXED,37.37105695228,126.72170433159,8.1249,22.3000,-0.3688,-0.2983,0.0300,-0.908838629,-0.130495900,213.736346026,0.4351,0.3021,0.5917,0.1155,0.0961,0.0864,0.0968,0.1008,5.0859,0f000001,0*b472baf5\n\tsystem status\tnormal 2 27.800000 0 0\trobot status\t76.994659\t102.855265\t8.124900\t-0.908839\t-0.130496\t-123.736346\t0.499000\t0.006000\n\t\n15:49:08.8\tlog_raw\tgps_raw\t#DUALANTENNAHEADINGA,USB3,0,49.5,FINESTEERING,2107,283766.800,02000000,d426,15824;INSUFFICIENT_OBS,NONE,-1.000000000,0.000000000,0.000000000,0.0,0.000000000,0.000000000,\"631T\",12,2,2,2,04,00,20,00*fb02124e\n\tsystem status\tnormal 2 27.800000 0 0\trobot status\t76.850709\t102.665468\t8.124000\t-0.711829\t-0.280100\t-123.897450\t0.406000\t-0.055000\n\t\n15:49:09.3\tlog_raw\tgps_raw\t#INSPVAXA,USB3,0,42.5,FINESTEERING,2107,283767.300,02000000,471d,15824;INS_ALIGNMENT_COMPLETE,INS_RTKFIXED,37.37105380440,126.72170132939,8.1248,22.3000,-0.4012,-0.3058,0.0222,-0.759918360,0.196787638,213.771684261,0.4356,0.3025,0.5930,0.1157,0.0960,0.0864,0.0969,0.1009,5.0866,0f000001,0*582355d6\n\tsystem status\tnormal 2 27.800000 0 0\trobot status\t76.728730\t102.505901\t8.124800\t-0.759918\t0.196788\t-123.771684\t0.501000\t0.015000\n\t\n15:49:09.8\tlog_raw\tgps_raw\t#DUALANTENNAHEADINGA,USB3,0,42.5,FINESTEERING,2107,283767.800,02000000,d426,15824;INSUFFICIENT_OBS,NONE,-1.000000000,0.000000000,0.000000000,0.0,0.000000000,0.000000000,\"631T\",11,2,2,2,04,00,20,00*0d855270\n\tsystem status\tnormal 2 27.800000 0 0\trobot status\t76.576795\t102.306238\t8.125300\t-0.442914\t0.234967\t-123.856430\t0.477000\t0.012000\n\t\n15:49:10.3\tlog_raw\tgps_raw\t#DUALANTENNAHEADINGA,USB3,0,49.5,FINESTEERING,2107,283768.300,02000000,d426,15824;INSUFFICIENT_OBS,NONE,-1.000000000,0.000000000,0.000000000,0.0,0.000000000,0.000000000,\"631T\",13,2,2,2,04,00,20,00*d65186ff\n\tsystem status\tnormal 2 27.800000 0 0\trobot status\t76.436672\t102.124531\t8.126600\t-0.426129\t0.683080\t-123.845040\t0.505000\t0.006000\n\t\n15:49:10.8\tlog_raw\tgps_raw\t#INSPVAXA,USB3,0,49.5,FINESTEERING,2107,283768.800,02000000,471d,15824;INS_ALIGNMENT_COMPLETE,INS_RTKFIXED,37.37104867092,126.72169640975,8.1299,22.3000,-0.3630,-0.2854,0.0072,-0.696189759,0.706458627,213.919013530,0.4366,0.3037,0.5940,0.1145,0.0950,0.0854,0.0970,0.1010,5.0873,0f000001,0*a94daabe\n\tsystem status\tnormal 2 27.800000 0 0\trobot status\t76.292956\t101.936168\t8.129900\t-0.696190\t0.706459\t-123.919014\t0.495000\t0.000000\n\t\n15:49:11.3\tlog_raw\tgps_raw\t#DUALANTENNAHEADINGA,USB3,0,49.0,FINESTEERING,2107,283769.300,02000000,d426,15824;INSUFFICIENT_OBS,NONE,-1.000000000,0.000000000,0.000000000,0.0,0.000000000,0.000000000,\"631T\",11,2,2,2,04,00,20,00*9a47621b\n\tsystem status\tnormal 2 27.800000 0 0\trobot status\t
